vi "Alpha 2.1.vi"() -> ()   [LabVIEW 2011]
uses:
  <vilib>/vision/Image Controls.llb/IMAQ Image.ctl
  <vilib>/vision/NI_Vision_Development_Module.lvlib
panel:
  in  "Browse":bool
  out "Image":T1(plugin-control)
  out "?":bool
  out "Path to Image":path
  in  "Image Type":T2 items=["Grayscale (U8)", "Grayscale (I16)", "Grayscale (SGL)", "Complex (CSG)", "RGB (U32)", "HSL (U32)", "RGB (U64)", "Grayscale (U16)"]
  in  "Lower":sgl(slide)=59.84694 scale=0.0..255.0
  in  "Upper":sgl(slide)=184.7449 scale=0.0..255.0
  in  "Stop Button":bool
  in  "Threshold":bool
  # "Lots and lots of bugs: -Image color looks strange\n                                  -No resize feature (due to laziness)\n                                  -Requires change of threshold to alter all settings"
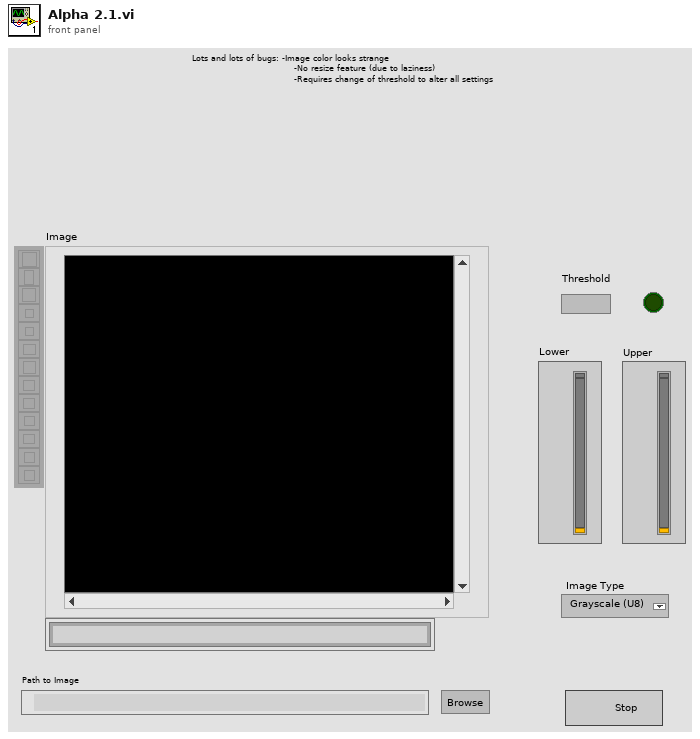
[diagram p1: front panel]
types:
  T1 = typedef "IMAQ Image.ctl" = refnum<image>
  T2 = typedef "Image Type" = u32
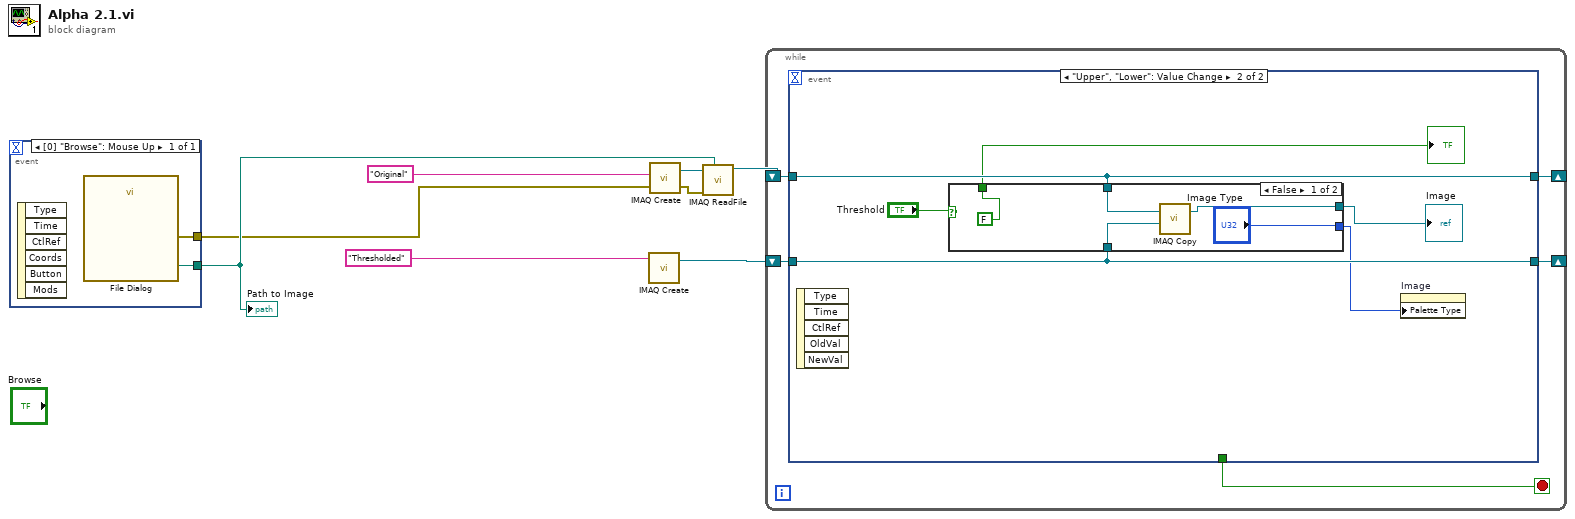
[diagram p0: block diagram]
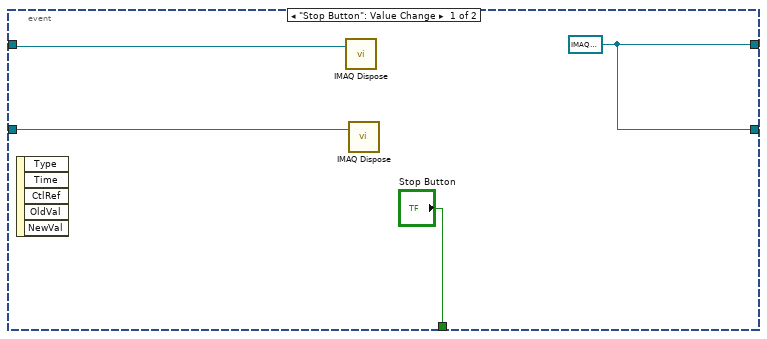
[diagram p2: hidden frame]
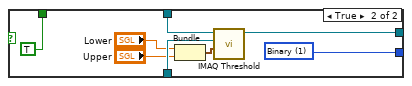
[diagram p3: hidden frame]
diagram:
  n1 = event shown="[0] \"Browse\": Mouse Up" {
    selector: _ -> [_]
    dyn-events: _ -> [_]
    timeout: _ -> [_]
    tunnel: [w10] -> w3
    tunnel: [w9] -> w2
    event "Browse": Mouse Up {
      n2 = event-data() -> ()  [unwired: 1 in, 6 out]
      n3 = call "File Dialog"() -> ("selected path"=w10:path, "error out"=w9:errorcluster)  [unwired: 12 in, 2 out]
    }
  }
  "Path to Image" <- w3
  n4 = call "IMAQ Create"("Image Name"="Thresholded") -> ("New Image"=w6:T1)  [unwired: 4 in, 1 out]
  n5 = call "IMAQ Create"("Image Name"="Original", "error in (no error)"=w2) -> ("New Image"=w5:T1, "error out"=w1:errorcluster)  [unwired: 3 in]
  n6 = call "IMAQ ReadFile"("File Path"=w3, "error in (no error)"=w1, "Image"=w5) -> ("Image Out"=w4:T1)  [unwired: 4 in, 4 out]
  n7 = while {
    shift-right: [w14] -> _
    shift-left: w4 -> [w15]
    shift-right: [w13] -> _
    shift-left: w6 -> [w12]
    stop <- w11 stop-if-true
    n8 = event shown="[1] \"Upper\", \"Lower\": Value Change" {
      selector: _ -> [_ _]
      dyn-events: _ -> [_ _]
      timeout: _ -> [_ _]
      tunnel: w15 -> [w17 w25]
      tunnel: [w16 w25] -> w14
      tunnel: [w16 w24] -> w13
      tunnel: w12 -> [w18 w24]
      tunnel: ["Stop Button" _] -> w11
      event "Stop Button": Value Change {
        w16 = T1 refnum ("New Image")
        n9 = event-data() -> ()  [unwired: 1 in, 5 out]
        n10 = call "IMAQ Dispose"("Image"=w17) -> ()  [unwired: 5 in, 1 out]
        n11 = call "IMAQ Dispose"("Image"=w18) -> ()  [unwired: 5 in, 1 out]
      }
      event "Upper", "Lower": Value Change {
        n12 = event-data() -> ()  [unwired: 1 in, 5 out]
        n13 = case shown="False" "Threshold" {
          tunnel: w25 -> [w30 w38]
          tunnel: w24 -> [w29 w37]
          tunnel: [w28 w36] -> w20
          tunnel: ["Image Type" w35] -> w21
          tunnel: [FALSE TRUE] -> w22
          frame False {
            n14 = call "IMAQ Copy"("Image Dst"=w29, "Image Src"=w30) -> ("Image Dst Out"=w28:T1)  [unwired: 4 in, 1 out]
          }
          frame True {
            w35 = u32 1 items=["Grayscale", "Binary", "Gradient", "Rainbow", "Temperature", "User Defined"] ("Palette:Palette Type")
            n15 = Bundle("Lower"="Lower", "Upper"="Upper") -> (w32:cluster{"Lower":sgl, "Upper":sgl})  [unwired: 1 in]
            n16 = call "IMAQ Threshold"("Range"=w32, "Image Dst"=w37, "Image Src"=w38) -> ("Image Dst Out"=w36:T1)  [unwired: 7 in, 1 out]
          }
        }
        "?" <- w22
        "Image" <- w20
        n17 = property on="Image" class="ImageControl"("Palette Type"=w21) -> ()  [unwired: 2 in, 2 out]
      }
    }
  }
